vi "Measure 2D Array.vi"(0 "eye scan in":refnum<class "niHighSpeedSerial Eye Scan v1 Host.lvclass">, 5 "instance":u8, 7 "requested number of new points":i32, 9 "timeout (100 ms)":dbl=0.1, 11 "error in":errorcluster) -> (2 "timed out?":bool, 3 "retrieved number of new points":i32, 4 "eye scan out":refnum<class "niHighSpeedSerial Eye Scan v1 Host.lvclass">, 6 "bit error ratio per point":dbl[][](array[numeric]), 8 "error count per point":u64[][](array[numeric]), 10 "sample count per point":u64[][](array[numeric]), 14 "done?":bool, 15 "error out":errorcluster)   [LabVIEW 2014, in "niHighSpeedSerial Eye Scan v1 Host.lvclass"]
doc: "Returns the Bit Error Rate, sample count, and error count on points that have been measured in 2D arrays.\nThis VI returns under the following conditions, whichever comes first:\n1) The <b>requested number of new points</b> are completed on each channel.\n2) The <b>timeout</b> is reached.\n3) The last point of the scan finishes measuring on all channels.\n\nIf you display the 2D Bit Error Rate output on an Intensity Graph, you can call Update Display on a Refnum of the Graph in order to properly format it.\n\n<B>Input Parameters</B>\n\n<B>eye scan in</B> Takes in a reference to your session from the previous VI.\n\n<B>instance</B> The instance of the channel to be used.\n\n<B>requested number of new points</B> The number of new points to return, assuming that timeout is not reached, the entire scan doesn't complete, and no errors occur.\n\n<B>timeout (100 ms)</B> The amount of time (in seconds) before timing timing out.\nSpecifying '-1' prevents 'timed out' from ever returning true.\n\n<B>error in</B> describes error conditions that occur before this node runs. This input provides standard 'error in' functionality.\n\n<B>Output Parameters</B>\n\n<B>retrieved number of new points</B> The number of new points that were retrieved in this call to Measure.\n\n<B>eye scan out</B> passes a reference to your session to the next VI.\n\n<B>bit error rate per point</B> is the calculated statistical bit error rate based on the number of error counts and sample counts received.\n\n<B>error count per point</B> is the number of errors received at each point.\n\n<B>sample count per point</B> is the number of samples measured at each point.\n\n<B>timed out?</B> returns true if at least 'timeout' amount of time has passed.\n\n<B>done?</B> returns true if the Eye Scan algorithm has completed measuring all points.\n\n<B>error out</B> contains error information. This output provides standard 'error out' functionality."
uses:
  <instrlib>/niHighSpeedSerial/Eye Scan/v1/Host/Eye Scan/niHighSpeedSerial Eye Scan v1 Host.lvclass
  <instrlib>/niHighSpeedSerial/Eye Scan/v1/Host/Eye Scan/niHighSpeedSerial Eye Scan v1 Host.lvclass/niHighSpeedSerial Eye Scan v1 Host.ctl
  <instrlib>/niHighSpeedSerial/Eye Scan/v1/Host/Impl/Eye Scan Point Iterator/niHighSpeedSerial Eye Scan Point Iterator v1 Host.lvclass
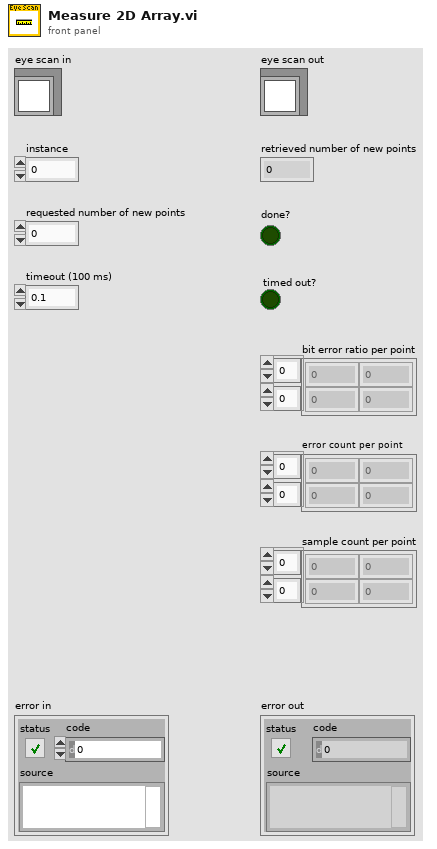
[diagram p1: front panel]
types:
  T1 = typedef "niHighSpeedSerial Eye Scan v1 Host.lvclass/Private Data.ctl" = cluster{"instruction target":refnum<class "niInstr Instruction Target v1 Host.lvclass">, "channels":T2[], "measure state":T3, "rx output divider":T4, "equalization mode":T5, "rx data width":T6, "BER floor":dbl, "number of points completed":i32, "rx output divider configured?":bool, "equalization mode configured?":bool, "rx data width configured?":bool}
  T2 = typedef "niHighSpeedSerial Eye Scan v1 Host.lvclass/Channel Data.ctl" = cluster{"instance":u8, "channel":refnum<class "niHighSpeedSerial Eye Scan Single Point v1 Host.lvclass">, "point iterator":refnum<class "niHighSpeedSerial Eye Scan Point Iterator v1 Host.lvclass">}
  T3 = typedef "niHighSpeedSerial Eye Scan v1 Host.lvclass/Measure State.ctl" = enum16{"Uninitialized", "Initialized", "Ready", "Measuring", "Finished", "Aborted"}
  T4 = typedef "niHighSpeedSerial Eye Scan Common v1 Host.lvlib/RX Output Divider.ctl" = enum16{"1", "2", "4", "8", "16"}
  T5 = typedef "niHighSpeedSerial Eye Scan Common v1 Host.lvlib/Equalization Mode.ctl" = enum16{"DFE", "LPM"}
  T6 = typedef "niHighSpeedSerial Eye Scan Common v1 Host.lvlib/Data Width.ctl" = enum16{"16 Bit", "20 Bit", "32 Bit", "40 Bit"}
  T7 = typedef "niHighSpeedSerial Eye Scan Common v1 Host.lvlib/Point.ctl" = cluster{"point offsets":T8, "sample count":u64, "error count":u64, "bit error ratio":dbl}
  T8 = typedef "niHighSpeedSerial Eye Scan Common v1 Host.lvlib/Point Offsets.ctl" = cluster{"horizontal offset":i16, "vertical offset":i8}
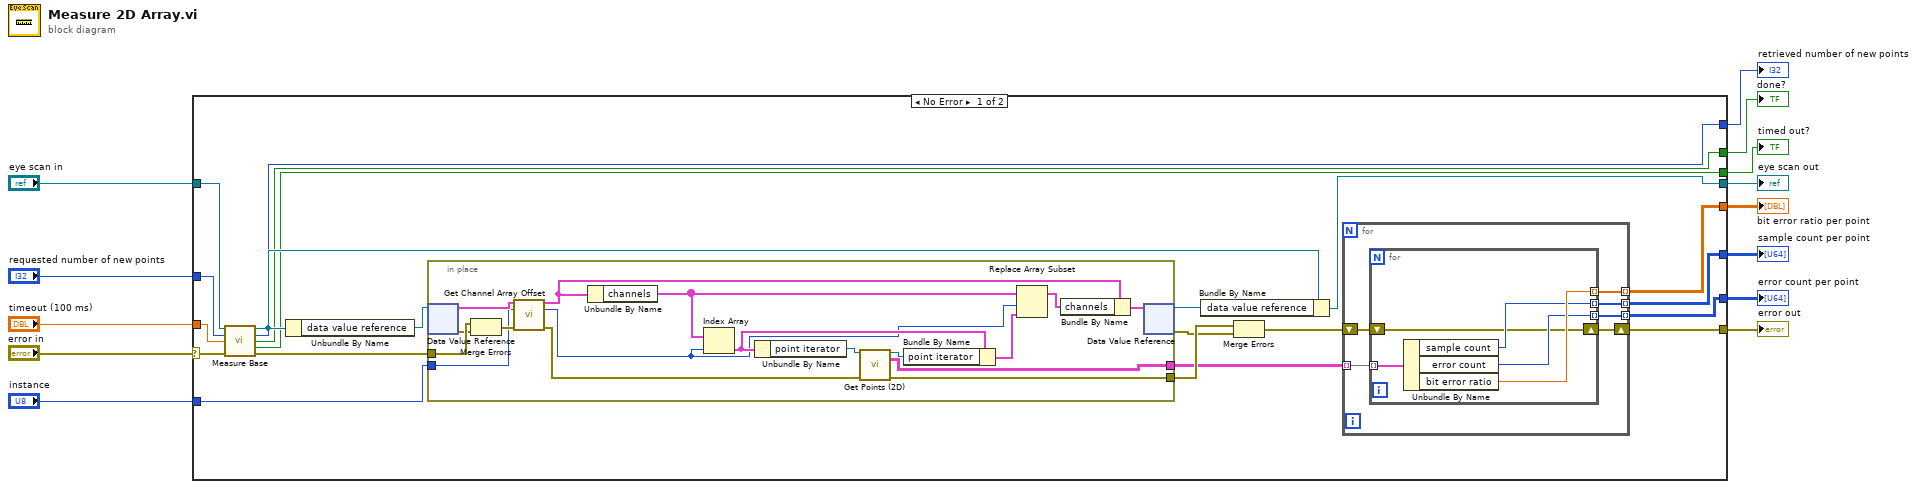
[diagram p0: block diagram]
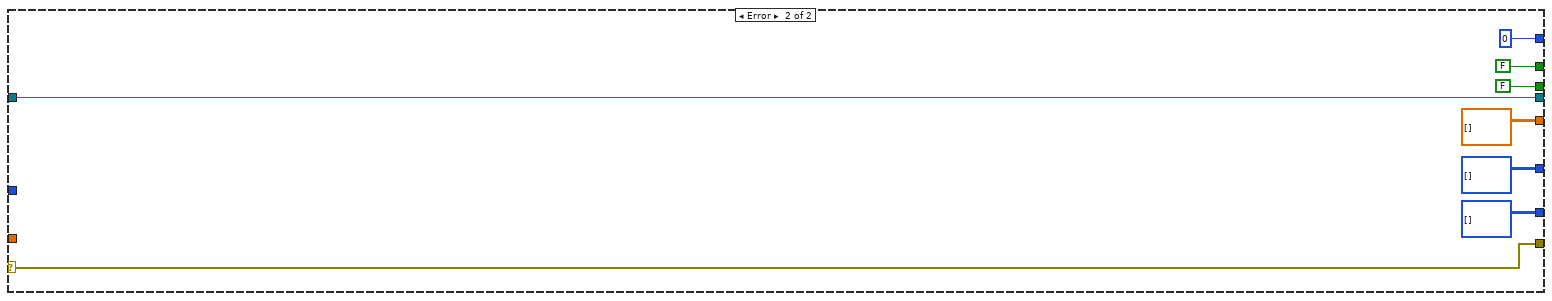
[diagram p2: hidden frame]
diagram:
  n1 = case shown="No Error" "error in" {
    selector: "error in" -> [w29 w70]
    tunnel: "eye scan in" -> [w31 w69]
    tunnel: [w32 w69] -> w11
    tunnel: "instance" -> [w26 _]
    tunnel: [w14 w70] -> w9
    tunnel: [w17 dbl[][] [] ("Bit Error Ratio Per Point")] -> w8
    tunnel: "timeout (100 ms)" -> [w27 _]
    tunnel: "requested number of new points" -> [w28 _]
    tunnel: [w16 u64[][] []] -> w1
    tunnel: [w24 FALSE] -> w5
    tunnel: [w18 u16[][] []] -> w2
    tunnel: [w25 0 ("Retrieved Number of New Points")] -> w4
    tunnel: [w23 FALSE ("Timed Out?")] -> w3
    frame No Error {
      n2 = call <instrlib>:"Measure Base.vi"("eye scan in"=w31, "requested number of new points"=w28, "timeout (100 ms)"=w27, "error in"=w29) -> ("eye scan out"=w30:refnum<class "niHighSpeedSerial Eye Scan v1 Host.lvclass">, "retrieved number of new points"=w25:i32, "last point measured?"=w24:bool, "timed out?"=w23:bool, "error out"=w20:errorcluster)  [unwired: 7 in]
      n3 = Unbundle By Name(w30) -> ("data value reference"=w34:refnum<data-value>)
      n4 = in-place {
        in-place-border: w26 -> [w47]
        in-place-border: w20 -> [w61]
        in-place-border: [w53] -> w22
        in-place-border: [w52] -> w19
        n5 = in-place-dvr #1(w34) -> (w48:T1, w60:errorcluster)
        n6 = Merge Errors(w61, w60) -> (w51:errorcluster)
        n7 = call <instrlib>:"Get Channel Array Offset.vi"("private data"=w48, "instance"=w47, "error in"=w51) -> ("private data out"=w49:T1, "channel array offset"=w46:i32, "error out"=w50:errorcluster)  [unwired: 10 in]
        n8 = Unbundle By Name(w49) -> ("channels"=w57:T2[])
        n9 = Index Array(array=w57, index=w46) -> (element=w59:T2)
        n10 = Unbundle By Name(w59) -> ("point iterator"=w62:refnum<class "niHighSpeedSerial Eye Scan Point Iterator v1 Host.lvclass">)
        n11 = call-dynamic "Get Points (2D).vi"("eye scan point iterator"=w62, "error in"=w50) -> ("eye scan point iterator out"=w58:refnum<class "niHighSpeedSerial Eye Scan Point Iterator v1 Host.lvclass">, "array of points"=w52:T7[][], "error out"=w53:errorcluster)  [unwired: 11 in]
        n12 = Bundle By Name(cluster=w59, "point iterator"=w58) -> (w56:T2)
        n13 = Replace Array Subset(array=w57, new element=w56, index=w46) -> (w55:T2[])
        n14 = Bundle By Name(cluster=w49, "channels"=w55) -> (w54:T1)
        n15 = in-place-dvr #1(w54) -> (w33:refnum<data-value>, w21:errorcluster)
      }
      n16 = Bundle By Name(cluster=w30, "data value reference"=w33) -> (w32:refnum<class "niHighSpeedSerial Eye Scan v1 Host.lvclass">)
      n17 = Merge Errors(w22, w21) -> (w15:errorcluster)
      n18 = for {
        tunnel: w19 -> [w40] mode=indexing
        tunnel: [w39] -> w16 mode=indexing
        tunnel: [w38] -> w17 mode=indexing
        shift-right: [w37] -> w14
        shift-left: w15 -> [w36]
        tunnel: [w35] -> w18 mode=indexing
        n19 = for {
          tunnel: w40 -> [w45] mode=indexing
          tunnel: [w43] -> w39 mode=indexing
          tunnel: [w42] -> w35 mode=indexing
          tunnel: [w44] -> w38 mode=indexing
          shift-right: [w41] -> w37
          shift-left: w36 -> [w41]
          n20 = Unbundle By Name(w45) -> ("sample count"=w43:u64, "error count"=w42:u64, "bit error ratio"=w44:dbl)
        }
      }
    }
    frame Error {
    }
  }
  "error out" <- w9
  "eye scan out" <- w11
  "done?" <- w5
  "retrieved number of new points" <- w4
  "timed out?" <- w3
  "bit error ratio per point" <- w8
  "error count per point" <- w2
  "sample count per point" <- w1
